vi "CreateProtectedEvents.vi"(8 "error in (no error)":errorcluster, 11 "JKI SMO.Example":refnum<class "SMO.Example.lvclass">) -> (0 "error out":errorcluster, 3 "JKI SMO.Example out":refnum<class "SMO.Example.lvclass">)   [LabVIEW 2013, in "SMO.Example.lvclass"]
doc: "---------------------------------------------------------------\nJKI State Machine Objects™\nhttp://jki.net/state-machine-objects/\nCopyright (C) 2005-2015, JKI <info@jki.net>\nALL RIGHTS RESERVED"
uses:
  SMO.Example.lvclass
  src/SMO/SMO.lvclass
  SMO.Example.lvclass/SMO.Example.ctl
  Typedefs/API Inputs--Cluster.ctl
  Typedefs/PumpState--Cluster.ctl
  Typedefs/ValveState--Cluster.ctl
panel:
  # "For instructions on how to use the JKI State Machine Objects, examples and video tutorials, visit:\nhttp://jki.net/state-machine-objects/\n\nJKI State Machine Objects™\nhttp://jki.net/state-machine-objects/\nCopyright (C) 2005-2015, JKI <info@jki.net>\nALL RIGHTS RESERVED"
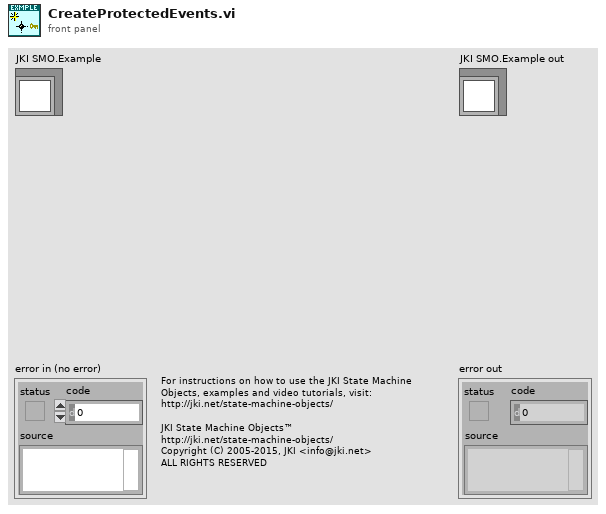
[diagram p1: front panel]
types:
  T1 = typedef "SMO.Example.lvclass/PrivateData--Ref.ctl" = refnum<data-value>
  T2 = typedef "SMO.Example.lvclass/ValveState--Cluster.ctl" = cluster{"State":bool}
  T3 = typedef "SMO.Example.lvclass/PumpState--Cluster.ctl" = cluster{"State":bool}
  T4 = typedef "SMO.Example.lvclass/API Inputs--Cluster.ctl" = cluster{"Data":string}
  T5 = typedef "SMO.Example.lvclass/PrivateData--Cluster.ctl" = cluster{"Configuration":T6, "Public Events":T7, "Protected Events":T8, "Flow 1":dbl, "Flow 2":dbl}
  T6 = typedef "SMO.Example.lvclass/Configuration--Cluster.ctl" = cluster{"Suffix":string}
  T7 = typedef "SMO.Example.lvclass/PublicEvents--Cluster.ctl" = cluster{"Data Changed":refnum<user-event>, "State Changed":refnum<user-event>}
  T8 = typedef "SMO.Example.lvclass/ProtectedEvents--Cluster.ctl" = cluster{"API_Template":refnum<user-event>, "PumpState":refnum<user-event>, "Valve State":refnum<user-event>}
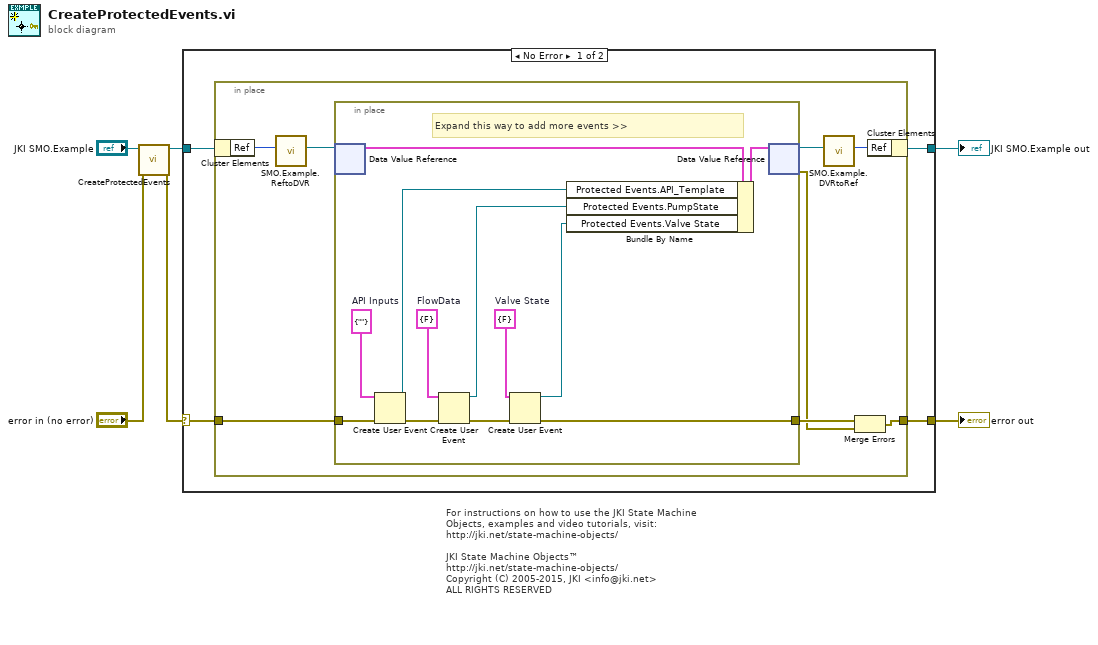
[diagram p0: block diagram]
diagram:
  # "For instructions on how to use the JKI State Machine Objects, examples and video tutorials, visit:\nhttp://jki.net/state-machine-objects/\n\nJKI State Machine Objects™\nhttp://jki.net/state-machine-objects/\nCopyright (C) 2005-2015, JKI <info@jki.net>\nALL RIGHTS RESERVED"
  n1 = call-parent "CreateProtectedEvents.vi"("error in (no error)"="error in (no error)", "SMO"="JKI SMO.Example") -> ("error out"=w1:errorcluster, "SMO out"=w3:refnum<class "SMO.Example.lvclass">)  [unwired: 8 in]
  n2 = case shown="No Error" w1 {
    selector: w1 -> [w8 w32]
    tunnel: [w7 w32] -> w5
    tunnel: [w9 w31] -> w6
    tunnel: w3 -> [w10 w31]
    frame No Error {
      n3 = in-place {
        in-place-border: w8 -> [w18]
        in-place-border: [w15] -> w7
        n4 = in-place-cluster #1(w10) -> ("Ref"=w14:u32)
        n5 = call "SMO.Example.ReftoDVR.vi"("Ref"=w14) -> ("Ref"=w13:T1)  [unwired: 10 in]
        n6 = in-place {
          in-place-border: w18 -> [w29]
          in-place-border: [w21] -> w17
          w20 = T2 {"State"=FALSE}  # Valve State
          w24 = T3 {"State"=FALSE}  # FlowData
          w27 = T4 {"Data"=""}  # API Inputs
          # "Expand this way to add more events >>"
          n7 = in-place-dvr #2(w13) -> (w28:T5)  [unwired: 1 out]
          n8 = Create User Event(user event datatype=w27, error in=w29) -> (user event=w26:refnum<user-event>, error out=w25:errorcluster)
          n9 = Create User Event(user event datatype=w24, error in=w25) -> (user event=w23:refnum<user-event>, error out=w22:errorcluster)
          n10 = Create User Event(user event datatype=w20, error in=w22) -> (user event=w19:refnum<user-event>, error out=w21:errorcluster)
          n11 = Bundle By Name(cluster=w28, "Protected Events.API_Template"=w26, "Protected Events.PumpState"=w23, "Protected Events.Valve State"=w19) -> (w30:T5)
          n12 = in-place-dvr #2(w30) -> (w12:T1, w16:errorcluster)
        }
        n13 = call "SMO.Example.DVRtoRef.vi"("Ref"=w12) -> ("Ref"=w11:u32)  [unwired: 10 in]
        n14 = Merge Errors(w17, w16) -> (w15:errorcluster)
        n15 = in-place-cluster #1("Ref"=w11) -> (w9:refnum<class "SMO.Example.lvclass">)
      }
    }
    frame Error {
    }
  }
  "error out" <- w5
  "JKI SMO.Example out" <- w6
